vi "Write Trigger.vi"(8 "error in (no error)":errorcluster, 10 "Trigger":u16(ring) items=["Internal", "External", "-", "-", "-", "-", "External Start"], 11 "CCDCamera in":refnum<class "Simulated_CCD_Camera.lvclass">) -> (0 "error out":errorcluster, 3 "CCDCamera out":refnum<class "Simulated_CCD_Camera.lvclass">)   [LabVIEW 2018, in "Simulated_CCD_Camera.lvclass"]
uses:
  Simulated_CCD_Camera.lvclass
  Simulated_CCD_Camera.lvclass/Simulated_CCD_Camera.ctl
  Interface/Interface.lvclass
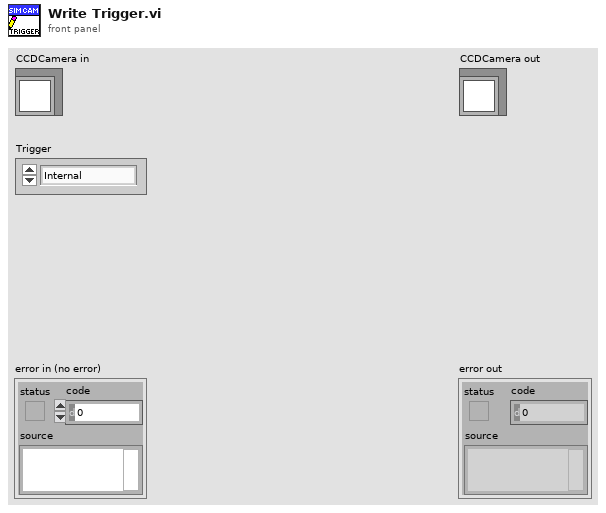
[diagram p1: front panel]
types:
  T1 = cluster{"EXPTIME":sgl, "PREAMP":u8, "READOUT_RATE":u8, "EM_MODE":u8, "EM_GAIN":u16, "BINNING":u16, "INITIAL_LINE":u16, "INITIAL_COLUMN":u16, "FINAL_LINE":u16, "FINAL_COLUMN":u16, "#FRAMES":u32, "#CUBES":u32, "TRIGGER_MODE":u16}
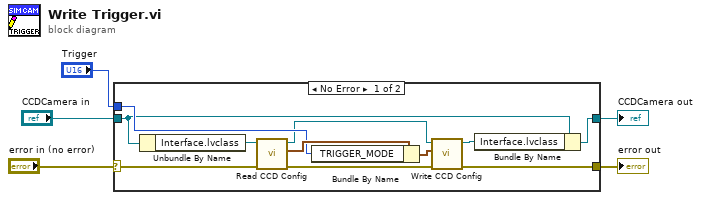
[diagram p0: block diagram]
diagram:
  n1 = case shown="No Error" "error in (no error)" {
    selector: "error in (no error)" -> [w7 w17]
    tunnel: [w9 w17] -> w4
    tunnel: [w12 w18] -> w2
    tunnel: "CCDCamera in" -> [w11 w18]
    tunnel: "Trigger" -> [w14 _]
    frame No Error {
      n2 = Unbundle By Name(w11) -> ("Interface.lvclass"=w13:refnum<class "Interface.lvclass">)
      n3 = call "Read CCD Config.vi"("error in (no error)"=w7, "Interface in"=w13) -> ("error out"=w8:errorcluster, "CCD Config"=w16:T1, "Interface out"=w6:refnum<class "Interface.lvclass">)  [unwired: 7 in]
      n4 = Bundle By Name(cluster=w16, "TRIGGER_MODE"=w14) -> (w15:T1)
      n5 = call "Write CCD Config.vi"("error in (no error)"=w8, "CCD Config"=w15, "Interface in"=w6) -> ("error out"=w9:errorcluster, "Interface out"=w10:refnum<class "Interface.lvclass">)  [unwired: 7 in]
      n6 = Bundle By Name(cluster=w11, "Interface.lvclass"=w10) -> (w12:refnum<class "Simulated_CCD_Camera.lvclass">)
    }
    frame Error {
    }
  }
  "error out" <- w4
  "CCDCamera out" <- w2
